vi "Memory.Pointer.Allocate (64-bit).vi"(8 "error in (no error)":errorcluster, 11 "size":i64 format="%d bytes") -> (0 "error out":errorcluster, 3 "Pointer out":refnum<class "Memory.Pointer.lvclass">)   [LabVIEW 2016, in "LabVIEW Memory Manager.lvlib" / "Memory.Pointer.lvclass"]
uses:
  Memory.Pointer.lvclass
  Memory.Pointer.lvclass/Memory.Pointer.ctl
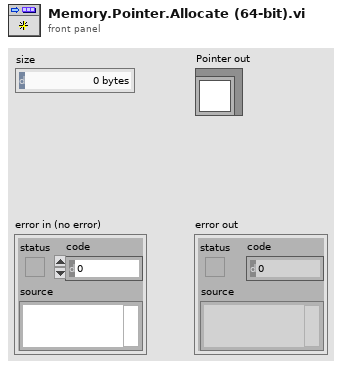
[diagram p1: front panel]
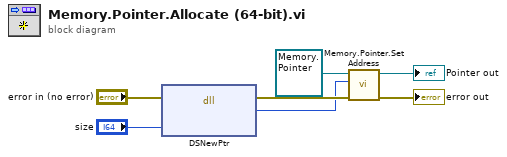
[diagram p0: block diagram]
diagram:
  n1 = dll-call lib="LabVIEW" fn="DSNewPtr"(error in="error in (no error)", "size"="size") -> (error out=w4:errorcluster, "pointer"=w3:u64)  [unwired: 3 in, 1 out]
  n2 = call "Memory.Pointer.Set Address.vi"("error in (no error)"=w4, "address"=w3, "Pointer in"=refnum<class "Memory.Pointer.lvclass"> refnum ("LabVIEW Memory Manager.lvlib:Pointer")) -> ("error out"=→"error out":errorcluster, "Pointer out"=→"Pointer out":refnum<class "Memory.Pointer.lvclass">)  [unwired: 7 in]
